vi "Interoperability.vi"() -> ()   [LabVIEW 2014]
panel:
  in  "STOP":bool
  out "Native":dbl
  out "MATLAB Node":dbl
  out "Formula Node":dbl
  in  "Max. Number":dbl=10.0
  # "SUMMATION OF N SEQUENCE"
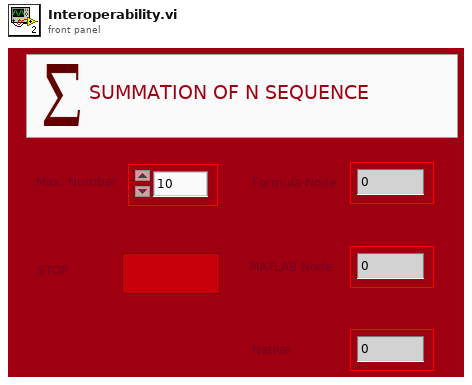
[diagram p1: front panel]
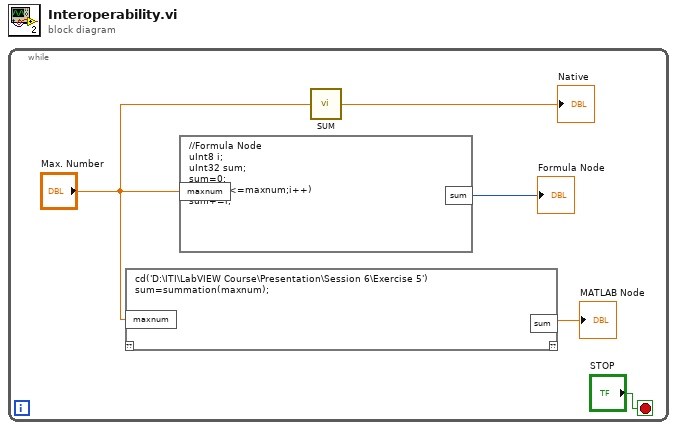
[diagram p0: block diagram]
diagram:
  n1 = while {
    stop <- "STOP" stop-if-true
    n2 = script code="cd('D:\\ITI\\LabVIEW Course\\Presentation\\Session 6\\Exercise 5')\nsum=summation(maxnum);"("maxnum"="Max. Number") -> ("sum"=→"MATLAB Node":dbl)  [unwired: 1 in, 1 out]
    n3 = formula code="//Formula Node\nuInt8 i;\nuInt32 sum;\nsum=0;\nfor(i=0;i<=maxnum;i++)\nsum+=i;"("maxnum"="Max. Number") -> ("sum"=→"Formula Node":u32)
    n4 = call "SUM.vi"("Max. Number"="Max. Number") -> ("Sum"=→"Native":dbl)
  }
